vi "File_GetConfigFilePath.vi"(5 "error in (no error)":errorcluster) -> (15 "Path":path, 19 "error out":errorcluster)   [LabVIEW 2014]
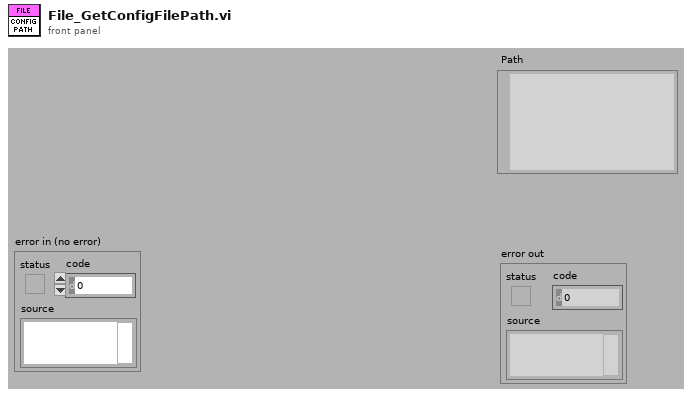
[diagram p1: front panel]
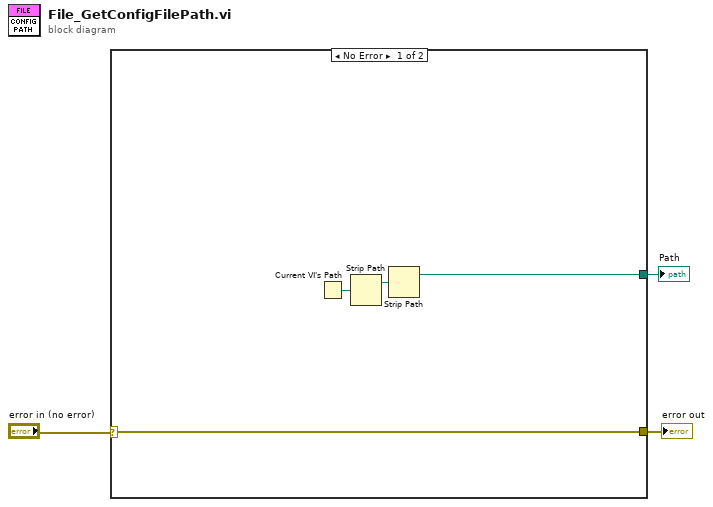
[diagram p0: block diagram]
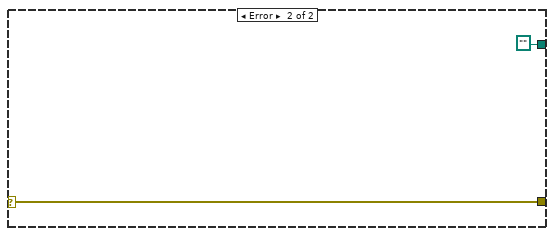
[diagram p2: hidden frame]
diagram:
  n1 = case shown="No Error" "error in (no error)" {
    selector: "error in (no error)" -> [w4 w9]
    tunnel: [w5 path ""] -> w2
    tunnel: [w4 w9] -> w1
    frame No Error {
      n2 = Current VI's Path() -> (path=w7:path)
      n3 = Strip Path(path=w7) -> (stripped path=w6:path)  [unwired: 1 out]
      n4 = Strip Path(path=w6) -> (stripped path=w5:path)  [unwired: 1 out]
    }
    frame Error {
    }
  }
  "Path" <- w2
  "error out" <- w1
